vi "Time elapsed FGV.vi"(10 "State":T1(ring), 11 "Time per floor":dbl=1.0 caption="Time Target (s)") -> (3 "Time elapsed":bool)   [LabVIEW 2019]
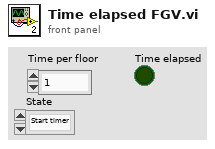
[diagram p1: front panel]
types:
  T1 = enum16{"Start timer", "Time elapsed", "Reset timer"}
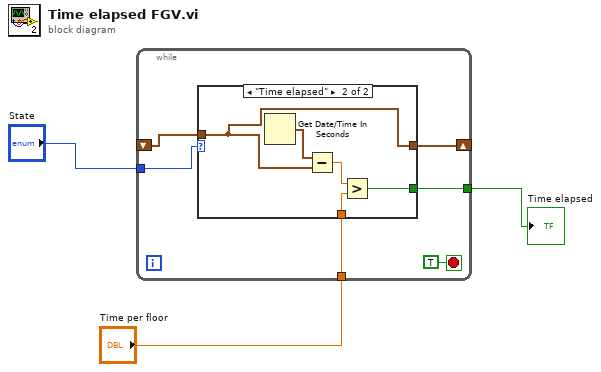
[diagram p0: block diagram]
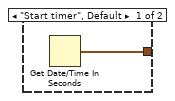
[diagram p2: hidden frame]
diagram:
  n1 = while {
    tunnel: "State" -> [w8]
    shift-right: [w7] -> _
    shift-left: _ -> [w6]
    tunnel: "Time per floor" -> [w5]
    tunnel: [w4] -> w3
    stop <- TRUE ("stop 2") stop-if-true
    n2 = case shown="\"Time elapsed\"" w8 {
      tunnel: [w10 w12] -> w7
      tunnel: w6 -> [_ w12]
      tunnel: w5 -> [_ w13]
      tunnel: [_ w11] -> w4
      frame "Start timer", Default {
        n3 = Get Date/Time In Seconds() -> (seconds since 1Jan1904=w10:timestamp)
      }
      frame "Time elapsed" {
        n4 = Get Date/Time In Seconds() -> (seconds since 1Jan1904=w15:timestamp)
        n5 = Subtract(x=w15, y=w12) -> (x-y=w14:dbl)
        n6 = Greater?(x=w14, y=w13) -> (0:w11:bool)
      }
    }
  }
  "Time elapsed" <- w3
